vi "CosimController.vi"() -> ()   [LabVIEW 2017]
uses:
  <vilib>/rvi/Analysis/control/PID/Typedef/niFpgaPID_PIGains.ctl
  FPGA/contState.ctl
  <vilib>/Simulation/Scripting/Companion Diagram/SimConfigNode/SimParams.ctl
  <vilib>/Simulation/Scripting/Companion Diagram/SimConfigNode/_simSolvers.ctl
  <vilib>/Simulation/Implementation/Shared/SIMSCR Execution Mode.ctl
  <vilib>/Simulation/Param Hierarchy/Typedefs/SIMPH Param Control Actions.ctl
  <vilib>/Simulation/Implementation/Shared/NILVSim_ParamChanged.vi
  <vilib>/Simulation/Implementation/Shared/NILVSIM_BeginStep.vi
  <vilib>/Utility/error.llb/Clear Errors.vi
  <vilib>/rvi/Emulation/niFpgaSctlEmulationGetInTimedLoop.vi
  <vilib>/Simulation/Utility/Implementation/SIM Halt.vi
  <vilib>/Simulation/Implementation/Shared/NILVSim_Manager.vi
  <vilib>/Simulation/Implementation/Shared/NILVSim_FinalizeModel.vi
  <vilib>/rvi/DataTransferAndStorage/Container/Common/niFpgaContainerExecOnDevCompGetState.vi
  <vilib>/rvi/Emulation/niFpgaEmulationIsFPGAContextNoSignature.vi
  <vilib>/rvi/DataTransferAndStorage/Container/Common/niFpgaContainerGetUniqueNameForEmu.vi
  <vilib>/rvi/Memory/Memory_Emulation/niFpgaMemoryEmulationCacheClearOnFirstRun.vi
  <vilib>/rvi/Memory/Memory_Emulation/nirvimemoryEmulationManagerCache_MakeExclusive.vi
  <vilib>/rvi/Memory/Memory_Emulation/niFpgaMemoryEmulationValidateCache.vi
  <vilib>/rvi/Memory/Memory_Emulation/nirvimemoryEmulationManagerCache_InsertValue.vi
  <vilib>/rvi/Memory/Memory_Emulation/nirvimemoryEmulationManagerCache_ReleaseExclusive.vi
  <vilib>/rvi/Memory/Memory_Emulation/nirvimemoryEmulationManagerCache_GetValue.vi
  <vilib>/rvi/Memory/Memory_Emulation/nirvimemoryEmulationManagerCache_SetValue.vi
  <vilib>/rvi/Emulation/niFpgaProcessEmulError.vi
  <vilib>/Simulation/Implementation/Shared/SIM Unbundle Sim Info.vi
  <vilib>/Simulation/Implementation/Shared/NILVSim_Initialize.vi
  FPGA/CurrentController.vi
  <vilib>/Simulation/Utility/Implementation/NILVSim Get Time and IsAcceptedStep.vi
  <vilib>/Simulation/Implementation/Shared/SIMSH Read Queue.vi
  <vilib>/Simulation/Implementation/Shared/NILVSim_GetModelError.vi
  <vilib>/Simulation/Implementation/Shared/SIM Bundle Sim Info.vi
  <vilib>/Simulation/Scripting/Companion Diagram/SimConfigNode/SimDog.xnode
  <vilib>/rvi/DataTransferAndStorage/Container/XNode/niFpgaContainer.xnode
  <vilib>/rvi/DataTransferAndStorage/Register/Emulation/niFpgaRegisterEmulationRefIn.vi
  <vilib>/Simulation/Implementation/XNodeFramework/SimXNode/SimX.xnode
  <vilib>/Simulation/EMI/Plugins/Multisim Design/MultisimEMICtrl.dll
  FPGA/BuckBoost.lvlib
  <vilib>/Simulation/Implementation/Shared/NI_SIM_Implementation.lvlib
panel:
  in  "state":T1
  in  "Halt?":bool
  out "Waveforms":dbl[][](graph)
  in  "gains":T2={"proportional gain"=1.0, "integral gain"=0.01} {"proportional gain" step=0.125}
  in  "reset":bool
  in  "I_setpt":sgl format="%#_13g"
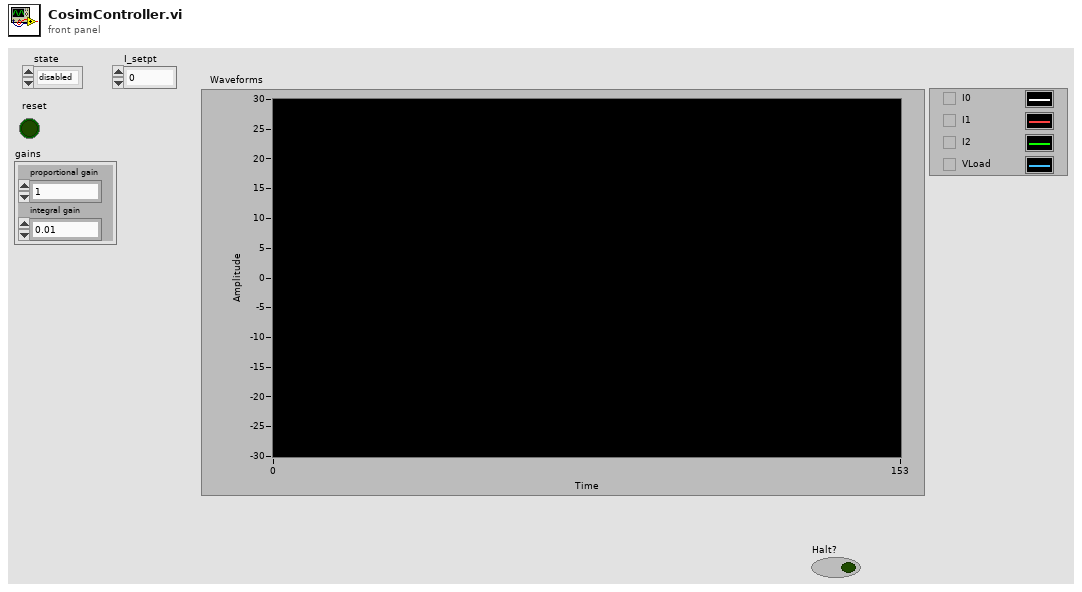
[diagram p1: front panel]
types:
  T1 = typedef "BuckBoost.lvlib/contState.ctl" = enum16{"disabled", "manual", "normal", "perturb"}
  T2 = typedef "niFpgaPID_PIGains.ctl" = cluster{"proportional gain":sgl, "integral gain":sgl}
  T3 = typedef "BuckBoost.lvlib/contSettings.ctl" = cluster{"numberOfInterleaves":refnum<k21>, "rampRate":refnum<k21>, "manualInput":refnum<k21>, "perturbAmp":refnum<k21>, "perturbAngleInc":refnum<k21>, "reset":refnum<k21>, "state":refnum<k21>, "gains":refnum<k21>, "Currents":refnum<k21>}
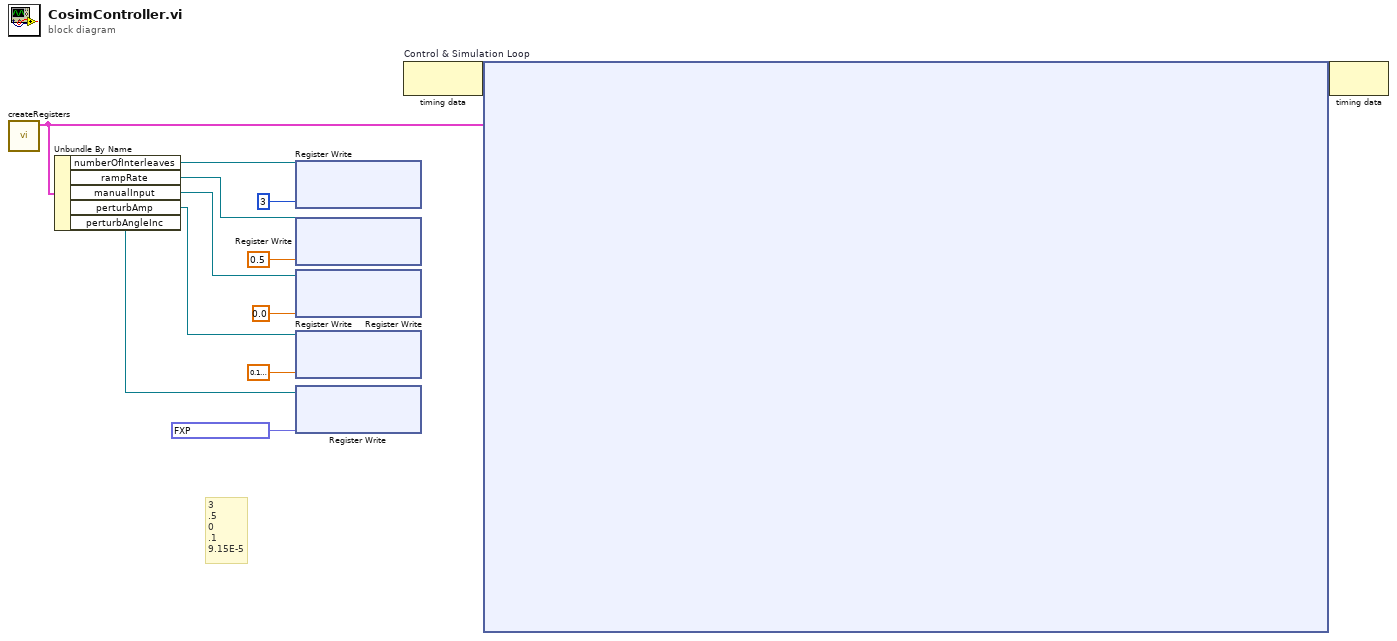
[diagram p0: block diagram]
diagram:
  # "3\n.5\n0\n.1\n9.15E-5"
  n1 = call "createRegisters.vi"() -> ("settingsReg"=w11:T3)  [unwired: 10 in, 1 out]
  n2 = Unbundle By Name(w11) -> ("numberOfInterleaves"=w10:refnum<k21>, "rampRate"=w9:refnum<k21>, "manualInput"=w8:refnum<k21>, "perturbAmp"=w7:refnum<k21>, "perturbAngleInc"=w6:refnum<k21>)
  n3 = xnode "Register Write"("Data"=u8 3, "Register In"=w10) -> ()  [unwired: 1 out]
  n4 = xnode "Register Write"("Data"=sgl 0.5, "Register In"=w9) -> ()  [unwired: 1 out]
  n5 = xnode "Register Write"("Data"=sgl 0.0, "Register In"=w8) -> ()  [unwired: 1 out]
  n6 = xnode "Register Write"("Data"=sgl 0.1, "Register In"=w7) -> ()  [unwired: 1 out]
  n7 = xnode "Register Write"("Data"=fxp<+/-,16,0> 1.52587890625e-05, "Register In"=w6) -> ()  [unwired: 1 out]
  n8 = node-c288() -> (w13:variant)  [unwired: 1 in]
  n9 = node-c254 "Control & Simulation Loop"(w13, w11) -> (w12:variant)
  n10 = node-c288(w12) -> ()  [unwired: 1 out]
